vi "Reset Host Buffer I16.vi"(7 "index":i32, 8 "error in":errorcluster, 11 "fpga session in":refnum<k20>) -> (0 "error out":errorcluster, 3 "fpga session out":refnum<k20>)   [LabVIEW 2017, in "Lock-In Amplifier Example Host.lvlib"]
uses:
  Lock-In Amplifier Example Host.lvlib
  fpga type.ctl
  <vilib>/Utility/error.llb/Error Cluster From Error Code.vi
  <vilib>/rvi/interface/nirviMethod/nirviMethod.xnode
  <vilib>/rvi/errors/niLvFpgaMergeErrorWithErrorCode.vi
  <vilib>/FPGAPlugInAG/Dynamic/niLvFpga_StopFifo_Dynamic.vi
  <vilib>/FPGAPlugInAG/Dynamic/niLvFpga_StartFifo_Dynamic.vi
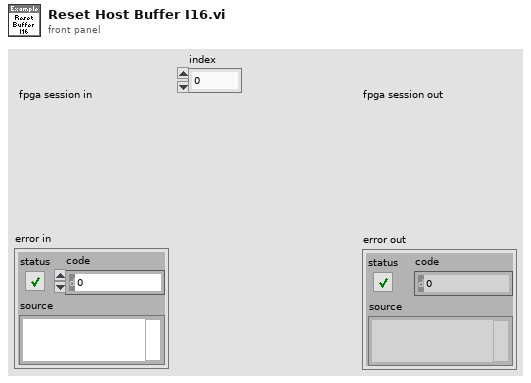
[diagram p1: front panel]
types:
  T1 = typedef "Lock-In Amplifier Example Host.lvlib/fpga type.ctl" = refnum<k20>
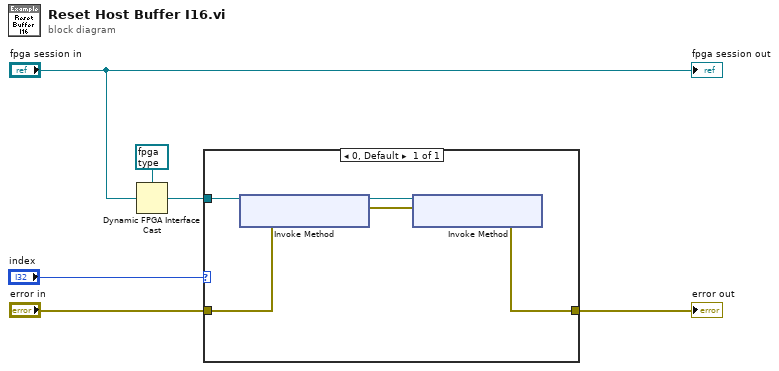
[diagram p0: block diagram]
diagram:
  n1 = Dynamic FPGA Interface Cast(Session In=T1 refnum ("fpga type"), Type="fpga session in") -> (Session Out=w4:T1)
  n2 = case shown="0, Default" "index" {
    tunnel: w4 -> [w11]
    tunnel: "error in" -> [w8]
    tunnel: [w7] -> w2
    frame 0, Default {
      n3 = xnode "Invoke Method"("FPGA VI Reference In"=w11, "error in"=w8) -> ("FPGA VI Reference Out"=w9:T1, "error out"=w10:errorcluster)
      n4 = xnode "Invoke Method"("FPGA VI Reference In"=w9, "error in"=w10) -> ("error out"=w7:errorcluster)  [unwired: 1 out]
    }
  }
  "error out" <- w2
  "fpga session out" <- "fpga session in"
